vi "getTimeStampString.vi"(8 "error in (no error)":errorcluster, 11 "Record in":refnum<class "Record.lvclass">) -> (0 "error out":errorcluster, 2 "Time Stamp String":string, 3 "Record out":refnum<class "Record.lvclass">)   [LabVIEW 2017]
uses:
  Record.lvclass
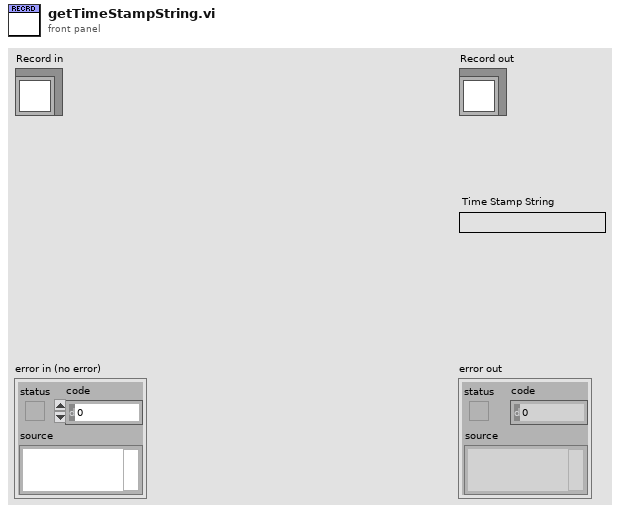
[diagram p1: front panel]
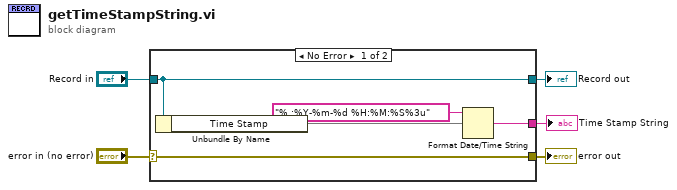
[diagram p0: block diagram]
diagram:
  n1 = case shown="No Error" "error in (no error)" {
    selector: "error in (no error)" -> [w10 w12]
    tunnel: [w10 w12] -> w4
    tunnel: [w8 w11] -> w2
    tunnel: "Record in" -> [w8 w11]
    tunnel: [w6 _] -> w1
    frame No Error {
      n2 = Unbundle By Name(w8) -> ("Time Stamp"=w7)
      n3 = Format Date/Time String(time format string (%c)="%.;%Y-%m-%d %H:%M:%S%3u", seconds (now)=w7) -> (date/time string=w6:string)  [unwired: 1 in]
    }
    frame Error {
    }
  }
  "error out" <- w4
  "Record out" <- w2
  "Time Stamp String" <- w1
